vi "Write Optimisation Strategy to string.vi"(1 "Value":dbl, 2 "Optimisation Strategy":T1) -> (0 "String":string)   [LabVIEW 2020, in "Run Utilities.lvlib" / "Optimiser Cell.lvclass"]
uses:
  Optimiser Cell.lvclass
  Optimisation Strategy.ctl
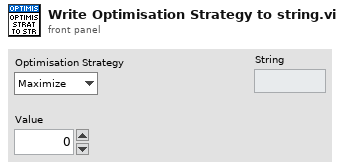
[diagram p1: front panel]
types:
  T1 = typedef "Run Utilities.lvlib/Optimiser Cell.lvclass/Optimisation Strategy.ctl" = enum16{"Maximize", "Minimize", "Value"}
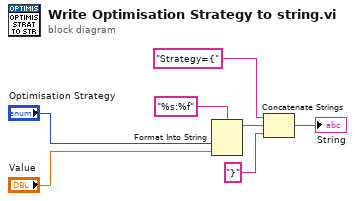
[diagram p0: block diagram]
diagram:
  n1 = Format Into String(format string="%s:%f", "Optimisation Strategy", "Value") -> (resulting string=w7:string)  [unwired: 2 in, 1 out]
  n2 = Concatenate Strings("Strategy={" ("string"), w7, "}" ("string")) -> (→"String":string)
